vi "Read Context.vi"(11 "Network Stream in":refnum<class "Network Stream.lvclass">) -> (2 "Context":string)   [LabVIEW 2020, in "Network Stream.lvclass"]
doc: "This VI returns the IP address for this endpoint of the network stream."
uses:
  <vilib>/NI/Actors/Network Endpoint Actors/Protocols/Network Stream Strategy/Network Stream/Network Stream.lvclass
  <vilib>/NI/Actors/Network Endpoint Actors/Protocols/Network Stream Strategy/Network Stream/Network Stream.lvclass/Network Stream.ctl
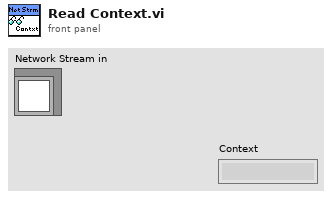
[diagram p1: front panel]
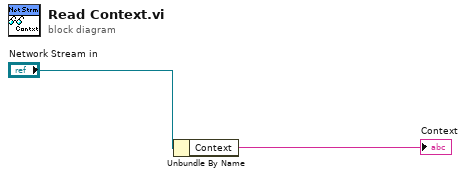
[diagram p0: block diagram]
diagram:
  n1 = Unbundle By Name("Network Stream in") -> ("Context"=→"Context":string)
